vi "SMSMagnet.ProcPeriodic.vi"(0 "i ref in":refnum<vi>, 3 "ms timeout (10000)":i32=10000, 5 "error in (no error)":errorcluster) -> (14 "i ref out":refnum<vi>, 17 "timed out":bool, 19 "error out":errorcluster)   [LabVIEW 2014, in "SMSMagnet.lvlib"]
doc: "This method serves to periodically do things like reading values from the HW. Methods that should be executed periodically should be called from THIS methode. Add code here."
uses:
  SMSMagnet.lvlib
  CSlibraries-extern/DimLVEvent/LVDimInterface/LVDimInterface.lvlib
  CSinstr.lib/SMSMagnetDriver/SMSMagnetDriver.lvlib
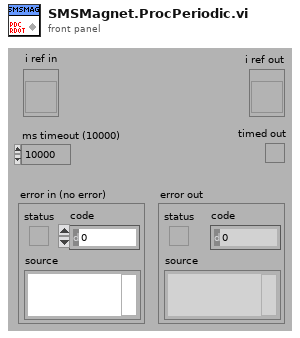
[diagram p1: front panel]
types:
  T1 = typedef "SMSMagnet.lvlib/SMSMagnet.i attribute.ctl" = cluster{"ActValueID":i32, "NomValueID":i32, "VISA resource name":refnum<visa-resource-name>, "ActValue":dbl, "VISAsem":T2}
  T2 = typedef "Semaphore RefNum" = refnum<k1>
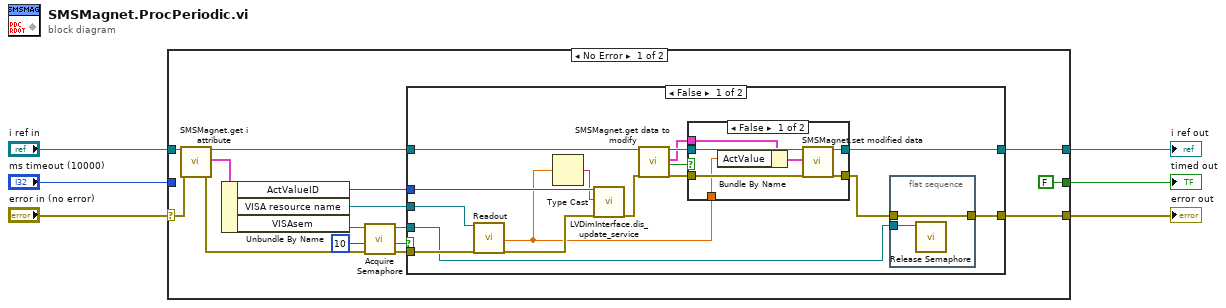
[diagram p0: block diagram]
diagram:
  n1 = case shown="No Error" "error in (no error)" {
    selector: "error in (no error)" -> [w19 w51]
    tunnel: [w13 w51] -> w5
    tunnel: "i ref in" -> [w20 w52]
    tunnel: [w14 w52] -> w3
    tunnel: [FALSE _] -> w2
    tunnel: "ms timeout (10000)" -> [_ _]
    frame No Error {
      n2 = call "SMSMagnet.get i attribute.vi"("i ref in"=w20, "error in (no error)"=w19) -> ("i ref out"=w15:refnum<vi>, "i attribute"=w18:T1, "error out"=w11:errorcluster)  [unwired: 15 in]
      n3 = Unbundle By Name(w18) -> ("ActValueID"=w17:i32, "VISA resource name"=w16:refnum<visa-resource-name>, "VISAsem"=w12:T2)
      n4 = call <vilib>:"Acquire Semaphore.vi"("error in (no error)"=w11, "ms timeout (-1)"=10, "semaphore"=w12) -> ("error out"=w10:errorcluster, "timed out"=w8:bool, "semaphore out"=w7:T2)  [unwired: 2 in]
      n5 = case shown="False" w8 {
        tunnel: w17 -> [w37 _]
        tunnel: w16 -> [w34 _]
        tunnel: w15 -> [w32 w50]
        tunnel: [w31 w50] -> w14
        tunnel: [w23 w49] -> w13
        tunnel: w10 -> [w25 w49]
        tunnel: w7 -> [w24 _]
        frame False {
          n6 = call "Readout.vi"("VISA resource name"=w34, "error in (no error)"=w25) -> ("Readback"=w26:dbl, "error out"=w35:errorcluster)  [unwired: 14 in, 2 out]
          n7 = Type Cast(x=w26) -> (*(type *) &x=w36:string)  [unwired: 1 in]
          n8 = call "LVDimInterface.dis_update_service.vi"("my_serviceID"=w37, "data"=w36, "error in (no error)"=w35) -> ("error out"=w30:errorcluster)  [unwired: 14 in, 2 out]
          n9 = call "SMSMagnet.get data to modify.vi"("i ref in"=w32, "error in (no error)"=w30) -> ("i ref out"=w33:refnum<vi>, "i attribute"=w27:T1, "timed out"=w28:bool, "error out"=w29:errorcluster)  [unwired: 14 in]
          n10 = case shown="False" w28 {
            tunnel: w33 -> [w46 w48]
            tunnel: [w45 w48] -> w31
            tunnel: w29 -> [w44 w47]
            tunnel: [w43 w47] -> w22
            tunnel: w27 -> [w42 _]
            tunnel: w26 -> [w40 _]
            frame False {
              n11 = Bundle By Name(cluster=w42, "ActValue"=w40) -> (w41:T1)
              n12 = call "SMSMagnet.set modified data.vi"("i ref in"=w46, "i attribute"=w41, "error in (no error)"=w44) -> ("i ref out"=w45:refnum<vi>, "error out"=w43:errorcluster)  [unwired: 15 in]
            }
            frame True {
            }
          }
          n13 = flat-sequence {
            tunnel: w24 -> [w39]
            tunnel: [w38] -> w23
            tunnel: w22 -> [w38]
            frame #0 {
              n14 = call <vilib>:"Release Semaphore.vi"("semaphore"=w39) -> ()  [unwired: 5 in, 2 out]
            }
          }
        }
        frame True {
        }
      }
    }
    frame Error {
    }
  }
  "error out" <- w5
  "i ref out" <- w3
  "timed out" <- w2
